vi "P13.vi"() -> ()   [LabVIEW 2018]
uses:
  <vilib>/vision/NI_Vision_Development_Module.lvlib
panel:
  out "error out":errorcluster
  in  "stop":bool
  in  "error in (no error)":errorcluster
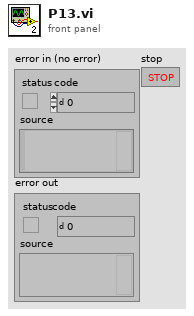
[diagram p1: front panel]
types:
  T1 = typedef "Image Type" = u32
  T2 = typedef "IMAQ Image.ctl" = refnum<image>
  T3 = typedef "ROI Descriptor" = cluster{"Global Rectangle":i32[], "Contours":cluster{"ID":enum32{"External", "Internal"}, "Type":u32, "Coordinates":i32[]}[]}
  T4 = typedef "IMAQ Rectangle" = cluster{"Left":i32, "Top":i32, "Right":i32, "Bottom":i32, "Rotation":dbl}
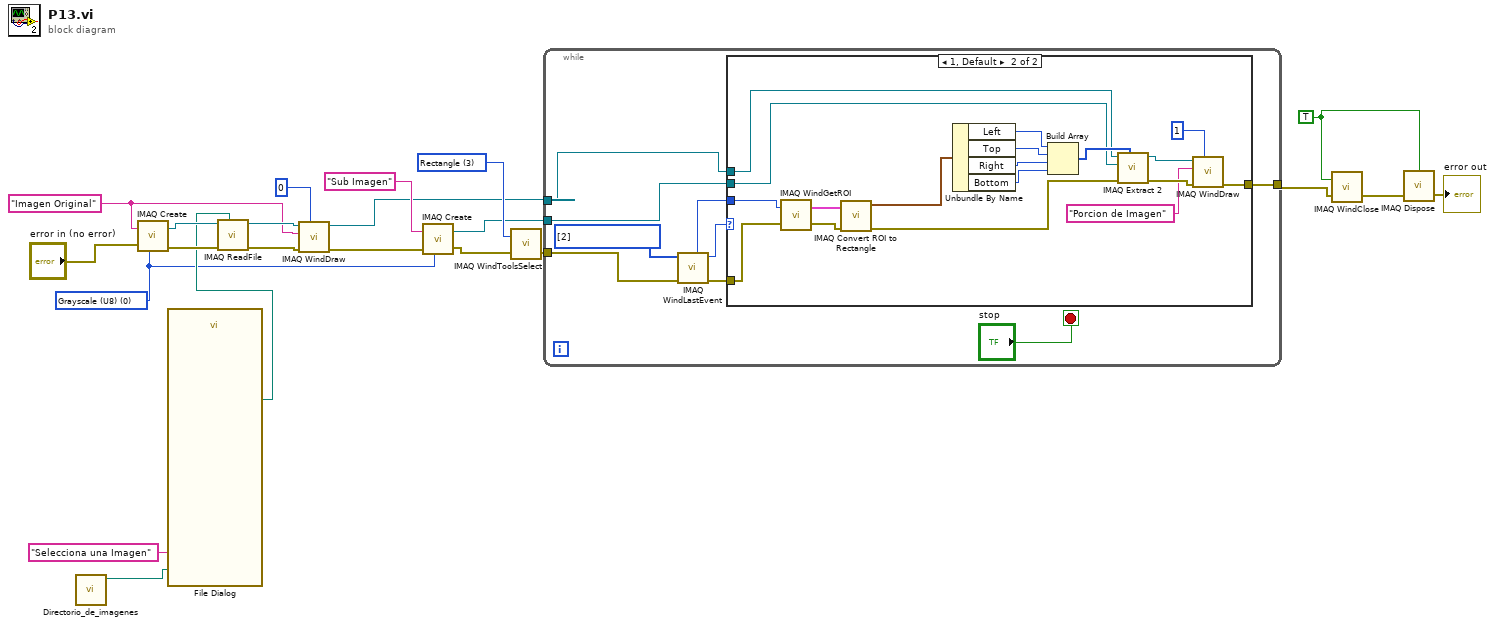
[diagram p0: block diagram]
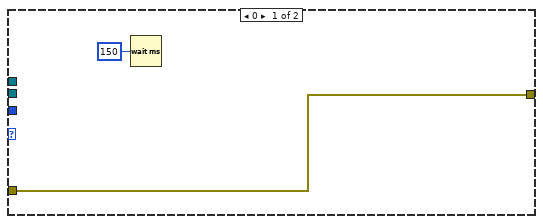
[diagram p2: hidden frame]
diagram:
  w1 = TRUE ("Close All Windows (False)")
  w8 = u32 3 items=["No Selection", "Point", "Line", "Rectangle", "Oval", "Polygon", "Freehand Region", "Annulus", "Zoom", "Pan", "Broken Line", "Freehand Line", "Rotated Rectangle"] ("Tool (Point)")
  w14 = "Imagen Original" ("Image Name")
  w12 = T1 0 items=["Grayscale (U8)", "Grayscale (I16)", "Grayscale (SGL)", "Complex (CSG)", "RGB (U32)", "HSL (U32)", "RGB (U64)", "Grayscale (U16)"] ("Image Type")
  n1 = call "Directorio_de_imagenes.vi"() -> ("stripped path"=w17:path)  [unwired: 11 in]
  n2 = call "IMAQ Create"("Image Name"=w14, "Image Type"=w12, "error in (no error)"="error in (no error)") -> ("New Image"=w20:T2, "error out"=w21:errorcluster)  [unwired: 2 in]
  n3 = call "File Dialog"("start path"=w17, "prompt"="Selecciona una Imagen") -> ("selected path"=w19:path)  [unwired: 10 in, 3 out]
  n4 = call <userlib>:"IMAQ ReadFile.vi"("File Path"=w19, "error in (no error)"=w21, "Image"=w20) -> ("error out"=w15:errorcluster, "Image Out"=w16:T2)  [unwired: 4 in, 3 out]
  n5 = call "IMAQ WindDraw"("Window Number (0...15)"=0, "error in (no error)"=w15, "Title"=w14, "Image"=w16) -> ("error out"=w10:errorcluster, "Image Out (duplicate)"=w7:T2)  [unwired: 6 in]
  n6 = call "IMAQ Create"("Image Name"="Sub Imagen", "Image Type"=w12, "error in (no error)"=w10) -> ("New Image"=w6:T2, "error out"=w11:errorcluster)  [unwired: 2 in]
  n7 = call "IMAQ WindToolsSelect"("Tool (Point)"=w8, "error in (no error)"=w11) -> ("error out"=w5:errorcluster)  [unwired: 3 in, 1 out]
  n8 = while {
    tunnel: w7 -> [w26]
    tunnel: w6 -> [w27]
    tunnel: w5 -> [w31]
    tunnel: [w24] -> w4
    stop <- "stop" stop-if-true
    w30 = i32[] [2] items=["No  event", "Click event", "Draw event", "Move event", "Size event", "Scroll event", "Activate event", "Close event", "Double click event"] ("Events list (all)")
    n9 = call "IMAQ WindLastEvent"("error in (no error)"=w31, "Events list (all)"=w30) -> ("error out"=w25:errorcluster, "Event"=w29:i32, "Window Number (0...15)"=w28:i32)  [unwired: 4 in, 3 out]
    n10 = case shown="1, Default" w29 {
      tunnel: w28 -> [_ w50]
      tunnel: w27 -> [_ w39]
      tunnel: w26 -> [_ w40]
      tunnel: w25 -> [w33 w51]
      tunnel: [w33 w34] -> w24
      frame 0 {
        n11 = Wait (ms)(milliseconds to wait=u32 150) -> ()  [unwired: 1 out]
      }
      frame 1, Default {
        n12 = call "IMAQ WindGetROI"("Window Number (0...15)"=w50, "error in (no error)"=w51) -> ("ROI Descriptor"=w48:T3, "error out"=w49:errorcluster)  [unwired: 3 in]
        n13 = call "IMAQ Convert ROI to Rectangle"("error in (no error)"=w49, "ROI Descriptor"=w48) -> ("error out"=w41:errorcluster, "Rectangle"=w47:T4)  [unwired: 7 in]
        n14 = Unbundle By Name(w47) -> ("Left"=w46:i32, "Top"=w45:i32, "Right"=w44:i32, "Bottom"=w43:i32)
        n15 = Build Array(w46, w45, w44, w43) -> (w42:i32[])
        n16 = call "IMAQ Extract 2"("Optional Rectangle"=w42, "error in (no error)"=w41, "Image Dst"=w39, "Image Src"=w40) -> ("error out"=w38:errorcluster, "Image Dst Out"=w37:T2)  [unwired: 6 in]
        n17 = call "IMAQ WindDraw"("Window Number (0...15)"=1, "error in (no error)"=w38, "Title"="Porcion de Imagen", "Image"=w37) -> ("error out"=w34:errorcluster)  [unwired: 6 in, 1 out]
      }
    }
  }
  n18 = call "IMAQ WindClose"("Close All Windows (False)"=w1, "error in (no error)"=w4) -> ("error out"=w3:errorcluster)  [unwired: 4 in]
  n19 = call "IMAQ Dispose"("All Images? (No)"=w1, "error in (no error)"=w3) -> ("error out"=→"error out":errorcluster)  [unwired: 4 in]
